vi "Detrend and Trend Estimation.vi"() -> ()   [LabVIEW 2023]
doc: "This example shows how to remove trends from a signal with the WA Detrend VI.\n\n<b>Instructions:</b>\n1) Run this VI.\n2) Change the <b>Wavelet</b> type and <b>Trend Level</b>.\n3) Observe the detrending performance in the <b>Detrend and Trend</b> graph."
uses:
  <vilib>/addons/Wavelet Analysis/typedefs.llb/WA Data.ctl
  <vilib>/addons/Wavelet Analysis/application.llb/WA Detrend (Waveform).vi
  <vilib>/addons/_Advanced Signal Processing/NI_AdvSigProcWA.lvlib
panel:
  in  "stop":bool
  out "Detrend and Trend":waveform(dbl)[](graph)
  out "Signal":waveform(dbl)(graph)
  in  "Wavelet":u16(ring) items=["db02"=0, "db03"=1, "db04"=2, "db05"=3, "db06"=4, "db07"=5, "db08"=6, "db09"=7, "db10"=8, "db11"=9, "db12"=10, "db13"=11, "db14"=12, "Haar"=13, "bior1_3"=14, "bior1_5"=15, "bior2_2"=16, "bior2_4"=17, "bior2_6"=18, "bior2_8"=19, "bior3_1"=20, "bior3_3"=21, "bior3_5"=22, "bior3_7"=23, "bior3_9"=24, "bior4_4 (FBI)"=25, "bior5_5"=38, "bior6_8"=39, "coif1"=26, "coif2"=27, "coif3"=28, "coif4"=29, "coif5"=30, "sym2"=31, "sym3"=32, "sym4"=33, "sym5"=34, "sym6"=35, "sym7"=36, "sym8"=37]
  in  "Threshold frequency":dbl=0.0125 min=0.0 max=1.0 step=0.0001 format="%.4f"
  # "Overview: Shows how to remove trends from a signal with the WA Detrend VI.\nRequirements: LabVIEW Full Development System, Advanced Signal Processing Toolkit\nInstructions: \n1. Run this VI.\n2. Change the Wavelet type and Trend Level.\n3. Observe the detrending performance in the Detrend and Trend graph.\n4. Click Stop to stop the VI."
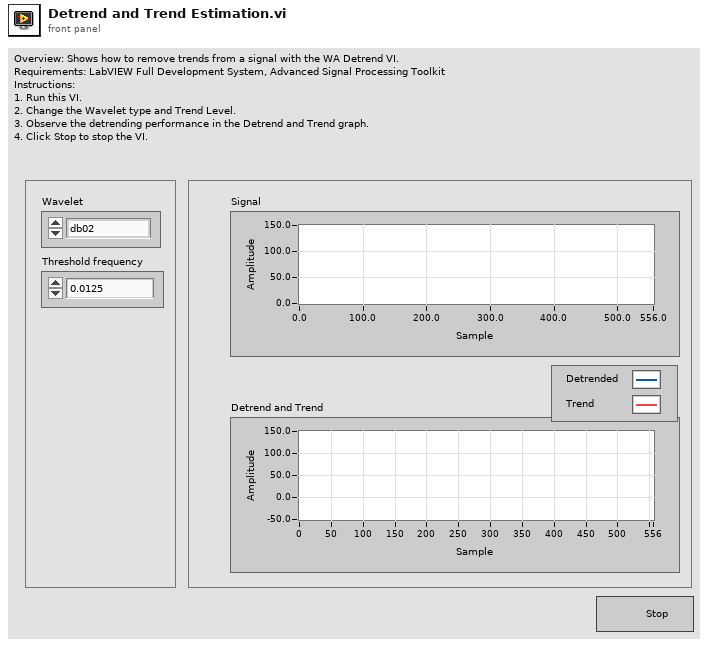
[diagram p1: front panel]
types:
  T1 = typedef "NI_AdvSigProcWA.lvlib/WA Data.ctl" = u16
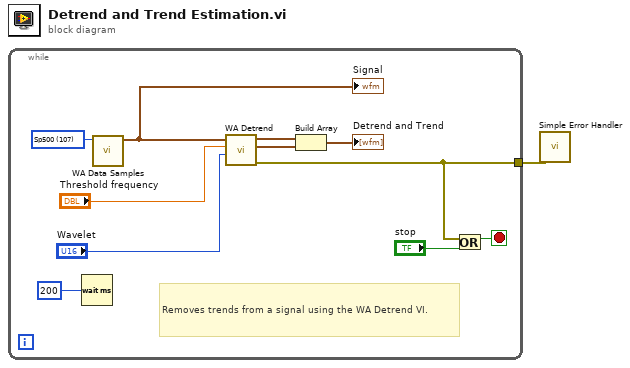
[diagram p0: block diagram]
diagram:
  n1 = while {
    tunnel: [w2] -> w1
    stop <- w5 stop-if-true
    w3 = T1 107 items=["1D Example Data"=100, "-"=101, "Doppler"=102, "HOP"=103, "TF Sine"=104, "Noisy Doppler"=105, "Sea Temperature"=106, "Sp500"=107, "Power Line"=108, "Engine Knocking"=109, "HeaviSine"=110, "Bumps"=111, "Blocks"=112, "Piece Regular"=113, "HypChirps"=114, "LinChirps"=115, "Chirps"=116, "Piece Polynomial"=117, "ECG"=131, "-"=118, "2D Example Data"=119, "-"=120, "Finger Print (Image)"=121, "Iris Flower (Image)"=122, "Mammogram (Image)"=123, "Lake (Image)"=127, "Two Can 1 (Image)"=132, "Two Can 2 (Image)"=133, "Camera Man (Image)"=134] ("data")
    # "Removes trends from a signal using the WA Detrend VI."
    n2 = Wait (ms)(milliseconds to wait=u32 200 ("millisecond multiple")) -> ()  [unwired: 1 out]
    n3 = call <vilib>:"WA Data Samples.vi"("data"=w3) -> ("signal"=w8:waveform(dbl))  [unwired: 10 out]
    "Signal" <- w8
    n4 = call-poly <vilib>:"WA Detrend.vi"("wavelet"="Wavelet", "threshold frequency"="Threshold frequency", "signal"=w8) -> ("error out"=w2:errorcluster, "trend signal"=w9:waveform(dbl), "detrended signal"=w10:waveform(dbl))  [unwired: 1 in, 5 out]
    n5 = Build Array(w10, w9) -> (→"Detrend and Trend":waveform(dbl)[])
    n6 = Or(x=w2, y="stop") -> (x .or. y?=w5:bool)
  }
  n7 = call <vilib>:"Simple Error Handler.vi"("error in (no error)"=w1) -> ()  [unwired: 1 in, 8 out]
